vi "Info Formatter.vi"(1 "Humidity (%)":fxp<+/-,64,32>, 2 "Temperature (°C)":fxp<+/-,64,32>) -> (0 "concatenated string":string)   [LabVIEW 2020]
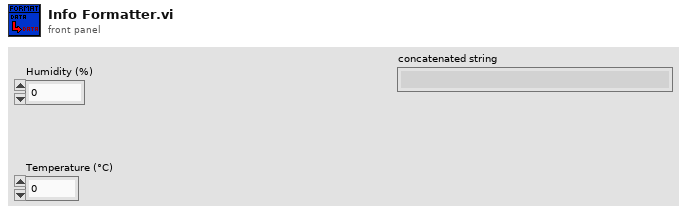
[diagram p1: front panel]
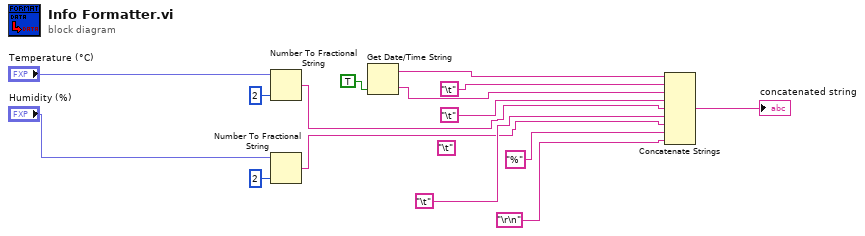
[diagram p0: block diagram]
diagram:
  (unwired) "\t"
  n1 = Number To Fractional String(number="Temperature (°C)", precision (6)=i16 2) -> (F-format string=w5:string)  [unwired: 2 in]
  n2 = Number To Fractional String(number="Humidity (%)", precision (6)=i16 2) -> (F-format string=w3:string)  [unwired: 2 in]
  n3 = Get Date/Time String(want seconds? (F)=TRUE) -> (date string=w12:string, time string=w14:string)  [unwired: 2 in]
  n4 = Concatenate Strings(w12, "\t", w14, "\t", w5, "\t", w3, "%", "\r\n") -> (→"concatenated string":string)
